vi "Project Item Recursion.vi"(8 "error in":errorcluster, 11 "TargetItem in":refnum<vi>) -> (0 "error out":errorcluster, 3 "TargetItem out":refnum<vi>[](array[refnum]))   [LabVIEW 2021, in "LV Scripting Utilities.lvlib"]
uses:
  LV Scripting Utilities.lvlib
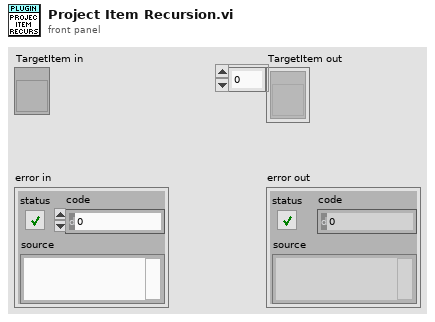
[diagram p1: front panel]
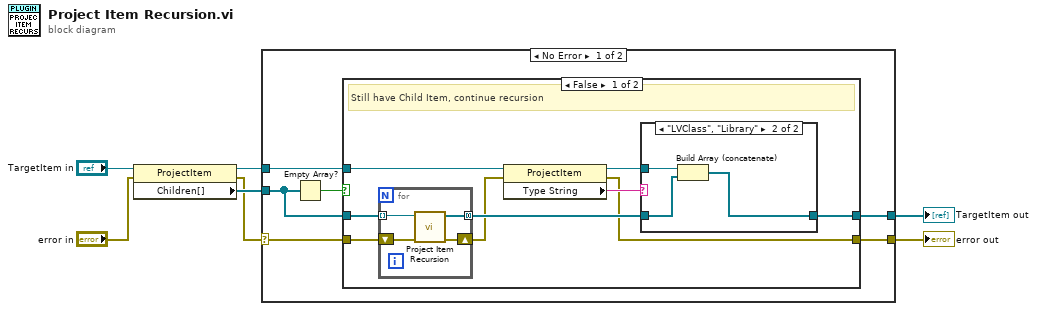
[diagram p0: block diagram]
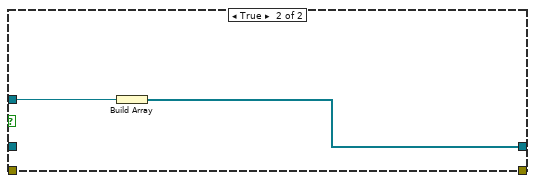
[diagram p3: hidden frame]
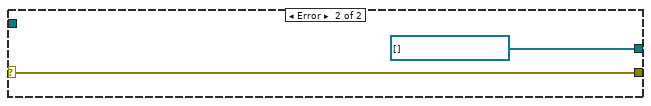
[diagram p4: hidden frame]
diagram:
  n1 = property class="ProjectItem"(reference="TargetItem in", error in="error in") -> (reference out=w3:refnum<vi>, error out=w1:errorcluster, "Children[]"=w2:refnum<vi>[])
  n2 = case shown="No Error" w1 {
    selector: w1 -> [w8 w33]
    tunnel: [w13 refnum<vi>[] [] ("TargetItem out")] -> w7
    tunnel: [w12 w33] -> w5
    tunnel: w3 -> [w10 _]
    tunnel: w2 -> [w9 _]
    frame No Error {
      n3 = Empty Array?(array=w9) -> (empty?=w11:bool)
      n4 = case shown="False" w11 {
        tunnel: [w17 w31] -> w13
        tunnel: w10 -> [w21 w32]
        tunnel: w9 -> [w22 _]
        tunnel: [w14 _] -> w12
        tunnel: w8 -> [w16 _]
        frame False {
          # "Still have Child Item, continue recursion"
          n5 = for {
            tunnel: w22 -> [w29] mode=indexing
            tunnel: [w30] -> w19 mode=concatenating
            shift-right: [w28] -> w15
            shift-left: w16 -> [w27]
            n6 = call "Project Item Recursion.vi"("error in"=w27, "TargetItem in"=w29) -> ("error out"=w28:errorcluster, "TargetItem out"=w30:refnum<vi>[])  [unwired: 8 in]
          }
          n7 = property class="ProjectItem"(reference=w21, error in=w15) -> (reference out=w18:refnum<vi>, error out=w14:errorcluster, "Type String"=w20:string)
          n8 = case shown="\"LVClass\", \"Library\"" w20 {
            tunnel: w19 -> [w23 w26]
            tunnel: w18 -> [_ w25]
            tunnel: [w23 w24] -> w17
            frame Default {
              # "Not target type of item"
            }
            frame "LVClass", "Library" {
              n9 = Build Array (concatenate)(w25, w26) -> (w24:refnum<vi>[])
            }
          }
        }
        frame True {
          n10 = Build Array(w32) -> (w31:refnum<vi>[])
        }
      }
    }
    frame Error {
    }
  }
  "TargetItem out" <- w7
  "error out" <- w5
